vi "Determine Actuator Position.vi"(8 "error in (no error)":errorcluster, 10 "Extended Lead":bool, 11 "Retracted Lead":bool=TRUE) -> (0 "error out":errorcluster, 2 "Actuator Position Enum":T1)   [LabVIEW 2016]
uses:
  Controls/Device Position Enum.ctl
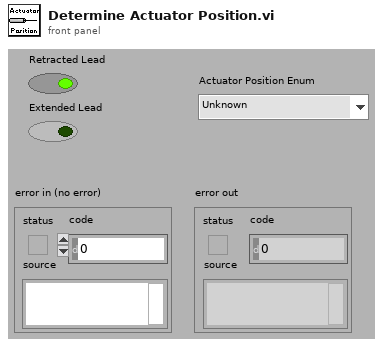
[diagram p1: front panel]
types:
  T1 = typedef "Device Position Enum.ctl" = enum16{"Unknown", "Actuator Is Moving", "Actuator Is Extended", "Actuator Is Retracted", "Disabled"}
  T2 = enum16{"Unknown", "Actuator Is Moving", "Actuator Is Extended", "Actuator Is Retracted"}
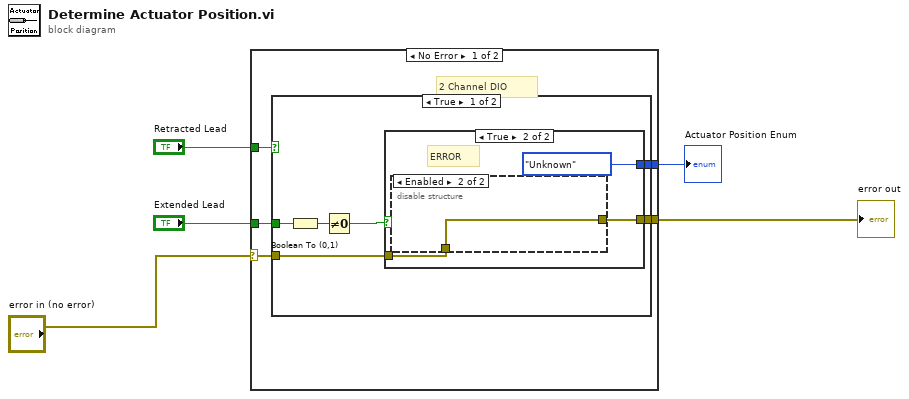
[diagram p0: block diagram]
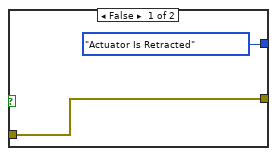
[diagram p2: hidden frame]
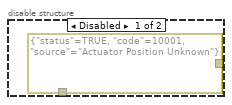
[diagram p3: hidden frame]
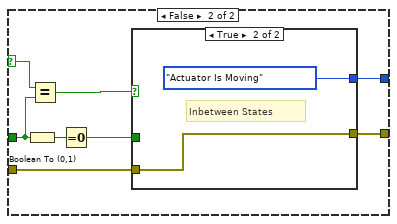
[diagram p4: hidden frame]
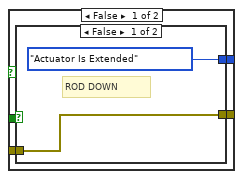
[diagram p5: hidden frame]
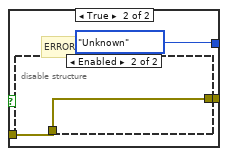
[diagram p6: hidden frame]
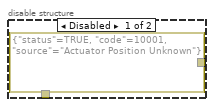
[diagram p7: hidden frame]
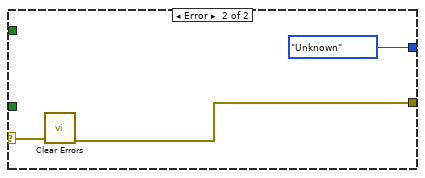
[diagram p8: hidden frame]
diagram:
  n1 = case shown="No Error" "error in (no error)" {
    selector: "error in (no error)" -> [w6 w47]
    tunnel: "Retracted Lead" -> [w10 _]
    tunnel: "Extended Lead" -> [w9 _]
    tunnel: [w8 w46] -> w3
    tunnel: [w7 Device_Position_Enum."Unknown"] -> w2
    frame No Error {
      # "2 Channel DIO"
      n2 = case shown="True" w10 {
        selector: w10 -> [_ w29]
        tunnel: w9 -> [w16 w28]
        tunnel: [w13 w26] -> w8
        tunnel: [w12 w25] -> w7
        tunnel: w6 -> [w11 w24]
        frame True {
          n3 = Boolean To (0,1)(Boolean=w16) -> (0, 1=w15:i16)
          n4 = Not Equal To 0?(x=w15) -> (x != 0?=w14:bool)
          n5 = case shown="True" w14 {
            tunnel: [w17 w21] -> w13
            tunnel: [Device_Position_Enum."Actuator Is Retracted" Device_Position_Enum."Unknown"] -> w12
            tunnel: w11 -> [w17 w19]
            frame False {
            }
            frame True {
              # "ERROR"
              n6 = disable-structure shown="Enabled" {
                disable-tunnel: [errorcluster {"status"=TRUE, "code"=10001, "source"="Actuator Position Unknown"} ("(No Error Constant)") w23] -> w21
                disable-tunnel: w19 -> [_ w23]
                frame Disabled {
                }
                frame Enabled {
                }
              }
            }
          }
        }
        frame False {
          n7 = Boolean To (0,1)(Boolean=w28) -> (0, 1=w31:i16)
          n8 = Equal?(x=w29, y=w28) -> (x = y?=w27:bool)
          n9 = Equal To 0?(x=w31) -> (x = 0?=w30:bool)
          n10 = case shown="True" w27 {
            tunnel: w30 -> [w35 _]
            tunnel: [w34 w43] -> w26
            tunnel: [w33 Device_Position_Enum."Actuator Is Moving"] -> w25
            tunnel: w24 -> [w32 w43]
            frame False {
              n11 = case shown="False" w35 {
                tunnel: [w36 w40] -> w34
                tunnel: [Device_Position_Enum."Actuator Is Extended" T2."Unknown"] -> w33
                tunnel: w32 -> [w36 w38]
                frame False {
                  # "ROD DOWN"
                }
                frame True {
                  # "ERROR"
                  n12 = disable-structure shown="Enabled" {
                    disable-tunnel: [errorcluster {"status"=TRUE, "code"=10001, "source"="Actuator Position Unknown"} ("(No Error Constant)") w42] -> w40
                    disable-tunnel: w38 -> [_ w42]
                    frame Disabled {
                    }
                    frame Enabled {
                    }
                  }
                }
              }
            }
            frame True {
              # "Inbetween States"
            }
          }
        }
      }
    }
    frame Error {
      n13 = call <vilib>:"Clear Errors.vi"("error in (no error)"=w47) -> ("error out"=w46:errorcluster)  [unwired: 1 in, 5 out]
    }
  }
  "error out" <- w3
  "Actuator Position Enum" <- w2
